vi "Emerson 5700 Reset Totalizers.vi"(7 "Reset all Totalizers. 2":T1=3 items=["Start/Stop Inventory 1"=367, "Start/Stop Inventory 2"=368, "Start/Stop all Totalizers and Inventories"=2, "Reset all Totalizers"=3, "Reset all Inventories"=4, "Reset Totalizer 1"=56, "Reset Totalizer 2"=57], 8 "Error In":errorcluster, 10 "Coil":bool=TRUE, 11 "address":string) -> (0 "Error Out":errorcluster)   [LabVIEW 2020]
uses:
  Type Definitions/Emerson 5700 Modbus Write Coils.ctl
  <vilib>/NI/Modbus Library/API/Wrapper/Create TCP Master.vi
  <vilib>/NI/Modbus Library/API/Master/Modbus Master.lvclass
  <vilib>/NI/Modbus Library/API/Wrapper/API Main.lvlib
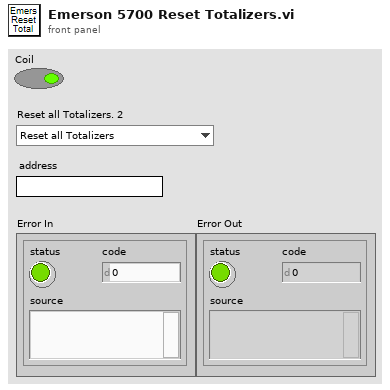
[diagram p1: front panel]
types:
  T1 = typedef "Emerson 5700 Modbus Write Coils.ctl" = u16
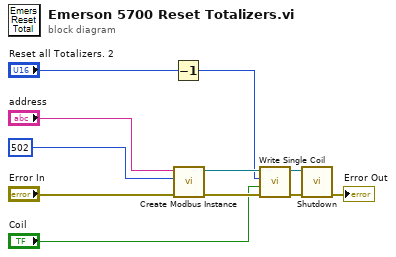
[diagram p0: block diagram]
diagram:
  n1 = Decrement(x="Reset all Totalizers. 2") -> (x-1=w4:T1)
  n2 = call-poly <vilib>:"Create Modbus Instance.vi"("error in"="Error In", "port (502)"=u16 502, "address"="address") -> ("error out"=w6:errorcluster, "TCP master instance"=w8:refnum<class "Modbus Master.lvclass">)  [unwired: 7 in]
  n3 = call-dynamic "Write Single Coil.vi"("error in"=w6, "coil to write"="Coil", "address"=w4, "Modbus master in"=w8) -> ("error out"=w7:errorcluster, "Modbus master out"=w9:refnum<class "Modbus Master.lvclass">)  [unwired: 6 in]
  n4 = call-dynamic "Shutdown.vi"("error in"=w7, "Modbus master in"=w9) -> ("error out"=→"Error Out":errorcluster)  [unwired: 9 in]
